vi "Write initial configuration.vi"(8 "error in (no error)":errorcluster, 11 "CCDCamera in":refnum<class "CCDCamera.lvclass">) -> (0 "error out":errorcluster, 3 "CCDCamera out":refnum<class "CCDCamera.lvclass">)   [LabVIEW 2018, in "CCDCamera.lvclass"]
doc: "Write the current operation mode to the camera"
uses:
  CCDCamera.lvclass
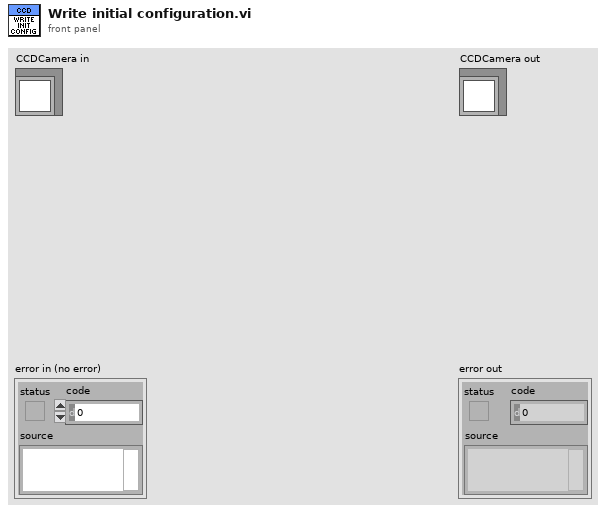
[diagram p1: front panel]
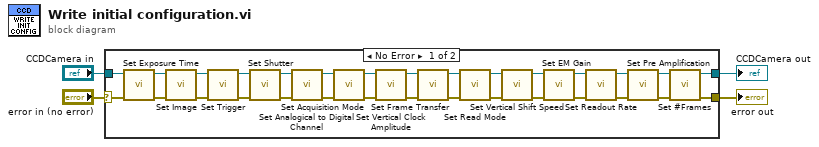
[diagram p0: block diagram]
diagram:
  n1 = case shown="No Error" "error in (no error)" {
    selector: "error in (no error)" -> [w6 w35]
    tunnel: "CCDCamera in" -> [w8 w36]
    tunnel: [w7 w36] -> w2
    tunnel: [w5 w35] -> w1
    frame No Error {
      n2 = call-dynamic "Set Exposure Time.vi"("error in (no error)"=w6, "CCDCamera in"=w8) -> ("error out"=w21:errorcluster, "CCDCamera out"=w34:refnum<class "CCDCamera.lvclass">)  [unwired: 8 in]
      n3 = call-dynamic "Set Image.vi"("error in (no error)"=w21, "CCDCamera in"=w34) -> ("error out"=w20:errorcluster, "CCDCamera out"=w33:refnum<class "CCDCamera.lvclass">)  [unwired: 8 in]
      n4 = call-dynamic "Set Trigger.vi"("error in (no error)"=w20, "CCDCamera in"=w33) -> ("error out"=w19:errorcluster, "CCDCamera out"=w32:refnum<class "CCDCamera.lvclass">)  [unwired: 8 in]
      n5 = call-dynamic "Set Shutter.vi"("error in (no error)"=w19, "CCDCamera in"=w32) -> ("error out"=w18:errorcluster, "CCDCamera out"=w31:refnum<class "CCDCamera.lvclass">)  [unwired: 8 in]
      n6 = call-dynamic "Set Analogical to Digital Channel.vi"("error in (no error)"=w18, "CCDCamera in"=w31) -> ("error out"=w17:errorcluster, "CCDCamera out"=w30:refnum<class "CCDCamera.lvclass">)  [unwired: 8 in]
      n7 = call-dynamic "Set Acquisition Mode.vi"("error in (no error)"=w17, "CCDCamera in"=w30) -> ("error out"=w16:errorcluster, "CCDCamera out"=w29:refnum<class "CCDCamera.lvclass">)  [unwired: 8 in]
      n8 = call-dynamic "Set Vertical Clock Amplitude.vi"("error in (no error)"=w16, "CCDCamera in"=w29) -> ("error out"=w15:errorcluster, "CCDCamera out"=w28:refnum<class "CCDCamera.lvclass">)  [unwired: 8 in]
      n9 = call-dynamic "Set Frame Transfer.vi"("error in (no error)"=w15, "CCDCamera in"=w28) -> ("error out"=w14:errorcluster, "CCDCamera out"=w27:refnum<class "CCDCamera.lvclass">)  [unwired: 8 in]
      n10 = call-dynamic "Set Read Mode.vi"("error in (no error)"=w14, "CCDCamera in"=w27) -> ("error out"=w13:errorcluster, "CCDCamera out"=w26:refnum<class "CCDCamera.lvclass">)  [unwired: 8 in]
      n11 = call-dynamic "Set Vertical Shift Speed.vi"("error in (no error)"=w13, "CCDCamera in"=w26) -> ("error out"=w12:errorcluster, "CCDCamera out"=w25:refnum<class "CCDCamera.lvclass">)  [unwired: 8 in]
      n12 = call-dynamic "Set EM Gain.vi"("error in (no error)"=w12, "CCDCamera in"=w25) -> ("error out"=w11:errorcluster, "CCDCamera out"=w24:refnum<class "CCDCamera.lvclass">)  [unwired: 8 in]
      n13 = call-dynamic "Set Readout Rate.vi"("error in (no error)"=w11, "CCDCamera in"=w24) -> ("error out"=w10:errorcluster, "CCDCamera out"=w23:refnum<class "CCDCamera.lvclass">)  [unwired: 8 in]
      n14 = call-dynamic "Set Pre Amplification.vi"("error in (no error)"=w10, "CCDCamera in"=w23) -> ("error out"=w9:errorcluster, "CCDCamera out"=w22:refnum<class "CCDCamera.lvclass">)  [unwired: 8 in]
      n15 = call-dynamic "Set #Frames.vi"("error in (no error)"=w9, "CCDCamera in"=w22) -> ("error out"=w5:errorcluster, "CCDCamera out"=w7:refnum<class "CCDCamera.lvclass">)  [unwired: 8 in]
    }
    frame Error {
    }
  }
  "error out" <- w1
  "CCDCamera out" <- w2
